vi "File Move (incoming to Archive).vi"(0 "source location of files":path, 1 "Files to Archive and FTP IN":string[][](array[string]), 5 "outgoing directory":path, 7 "redundant archive location":path, 9 "Archive 2 valid path":bool, 11 "error IO IN":errorcluster) -> (15 "Array of errors from file copy and or move":errorcluster[][](array[cluster]))   [LabVIEW 2011]
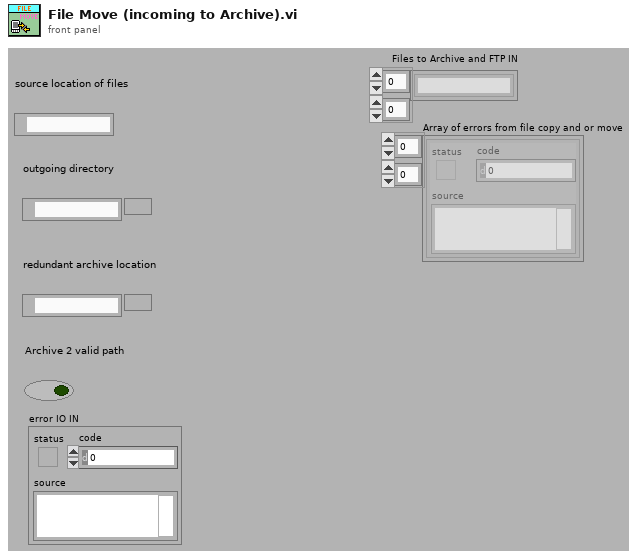
[diagram p1: front panel]
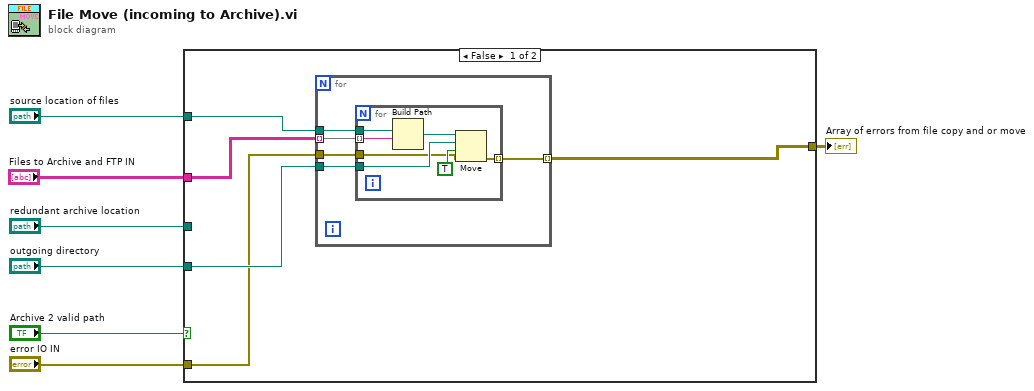
[diagram p0: block diagram]
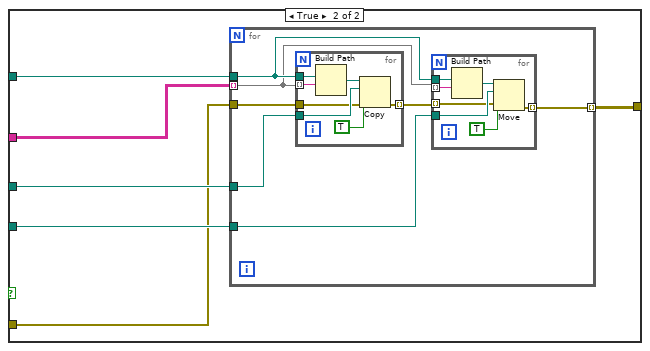
[diagram p2: hidden frame]
diagram:
  n1 = case shown="False" "Archive 2 valid path" {
    tunnel: "source location of files" -> [w10 w27]
    tunnel: "outgoing directory" -> [w12 w29]
    tunnel: "redundant archive location" -> [_ w30]
    tunnel: [w8 w28] -> w1
    tunnel: "error IO IN" -> [w9 w26]
    tunnel: "Files to Archive and FTP IN" -> [w11 w25]
    frame False {
      n2 = for {
        tunnel: w11 -> [w17] mode=indexing
        tunnel: w10 -> [w16]
        tunnel: w9 -> [w15]
        tunnel: w12 -> [w14]
        tunnel: [w13] -> w8 mode=indexing
        n3 = for {
          tunnel: w17 -> [w23] mode=indexing
          tunnel: w16 -> [w24]
          tunnel: w14 -> [w21]
          tunnel: w15 -> [w19]
          tunnel: [w18] -> w13 mode=indexing
          n4 = Build Path(base path=w24, name or relative path=w23) -> (appended path=w22:path)
          n5 = Move(source path=w22, error in=w19, 9:TRUE ("overwrite (F)"), 10:w21) -> (error out=w18:errorcluster)  [unwired: 1 in, 2 out]
        }
      }
    }
    frame True {
      n6 = for {
        tunnel: w30 -> [w37]
        tunnel: w29 -> [w35]
        tunnel: [w34] -> w28 mode=indexing
        tunnel: w27 -> [w33]
        tunnel: w26 -> [w32]
        tunnel: w25 -> [w31] mode=indexing
        n7 = for {
          tunnel: w31 -> [w43] mode=indexing
          tunnel: w33 -> [w44]
          tunnel: w37 -> [w41]
          tunnel: w32 -> [w39]
          tunnel: [w38] -> w36 mode=indexing
          n8 = Build Path(base path=w44, name or relative path=w43) -> (appended path=w42:path)
          n9 = Copy(8:w39, 9:TRUE ("overwrite (F)"), 10:w41, 11:w42) -> (0:w38:errorcluster)  [unwired: 1 in, 2 out]
        }
        n10 = for {
          tunnel: w31 -> [w50] mode=indexing
          tunnel: w33 -> [w51]
          tunnel: w35 -> [w48]
          tunnel: w36 -> [w46] mode=indexing
          tunnel: [w45] -> w34 mode=indexing
          n11 = Build Path(base path=w51, name or relative path=w50) -> (appended path=w49:path)
          n12 = Move(source path=w49, error in=w46, 9:TRUE ("overwrite (F)"), 10:w48) -> (error out=w45:errorcluster)  [unwired: 1 in, 2 out]
        }
      }
    }
  }
  "Array of errors from file copy and or move" <- w1
